vi "Receive DS Packet.vi"(0 "Recv Socket":refnum<k16>, 5 "Log User Data":bool) -> (2 "New Dashboard Data":bool, 3 "Battery":sgl, 4 "Error Strings":string, 6 "Driver Station":T1, 8 "Robot IP Address":string="10.0.0.2", 10 "Status":T3, 12 "Camera IP Address":string="10.0.0.2", 13 "Low Priority User Data":string, 14 "High Priority User Data":string, 15 "Error":T2)   [LabVIEW 2012]
uses:
  DStoPCPacketTypeDef.ctl
panel:
  out "CRC":string
  out "Team ID":u16
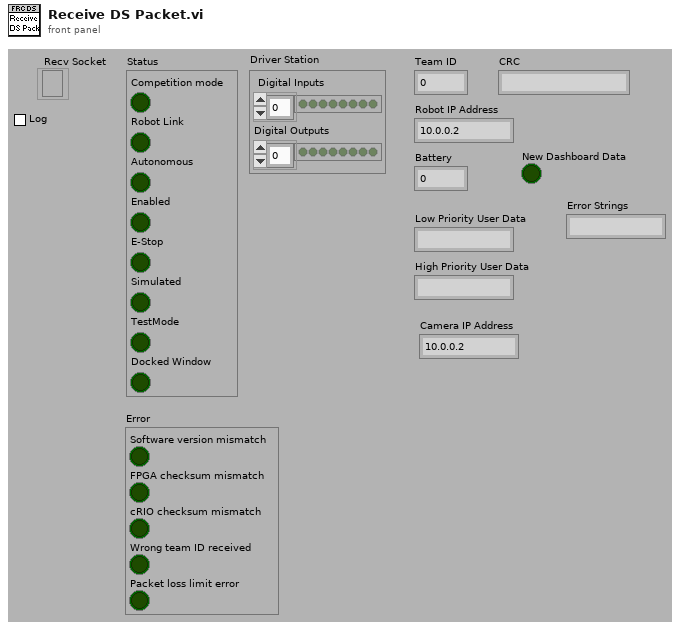
[diagram p1: front panel]
types:
  T1 = cluster{"Digital Inputs":bool[], "Digital Outputs":bool[]}
  T2 = cluster{"Software version mismatch":bool, "FPGA checksum mismatch":bool, "cRIO checksum mismatch":bool, "Wrong team ID received":bool, "Packet loss limit error":bool}
  T3 = cluster{"Competition mode":bool, "Robot Link":bool, "Autonomous":bool, "Enabled":bool, "E-Stop":bool, "Simulated":bool, "TestMode":bool, "Docked Window":bool}
  T4 = typedef "DStoPCPacketTypeDef.ctl" = cluster{"Packet Index":u16, "Digital Inputs":u8, "Digital Out":u8, "Battery":u16, "Status":u8, "Error":u8, "Team ID":u16, "VersionMonth1":u8, "VersionMonth2":u8, "VersionDay1":u8, "VersionDay2":u8, "VersionYear1":u8, "VersionYear2":u8, "Revision1":u8, "Revision2":u8, "Robot IP":u32, "UnusedBuffer 2":u8, "ExtraModeFlags":u8, "Reply Packet #":u16}
  T5 = cluster{"Boolean array":bool[], "Boolean array":bool[]}
  T6 = cluster{"Boolean array[0]":bool, "Boolean array[1]":bool, "Boolean array[2]":bool, "Boolean array[3]":bool, "Boolean array[4]":bool, "Boolean array[5]":bool, "Boolean array[6]":bool, "Boolean array[7]":bool}
  T7 = cluster{"Boolean array[0]":bool, "Boolean array[1]":bool, "Boolean array[4]":bool, "Boolean array[5]":bool, bool, bool, bool, bool}
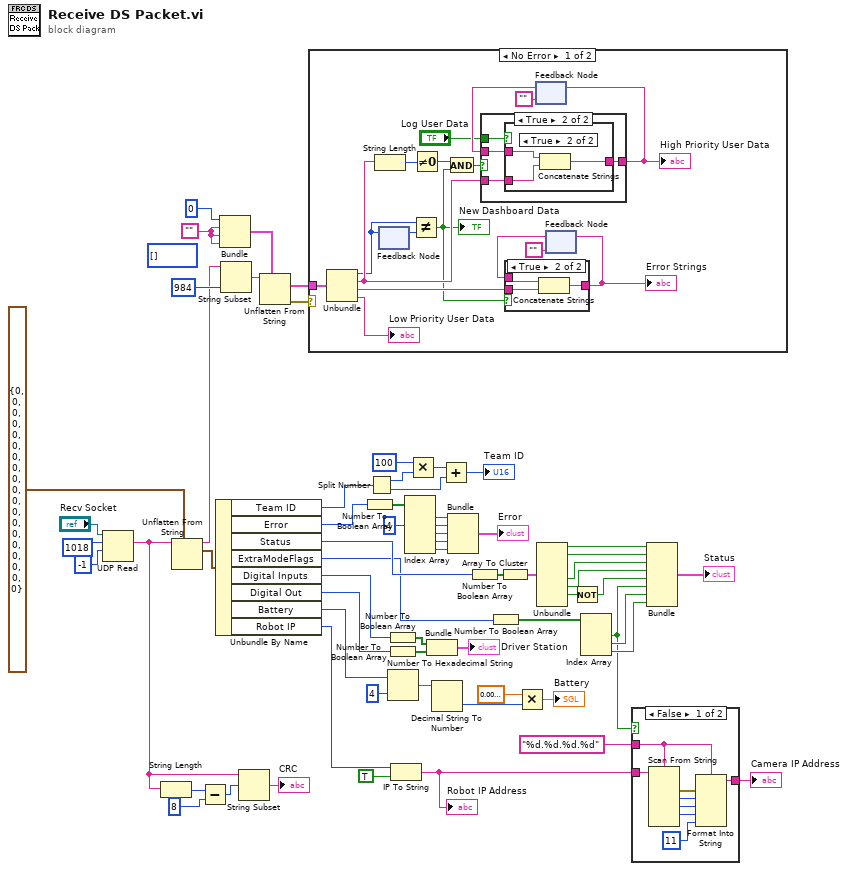
[diagram p0: block diagram]
diagram:
  (unwired) u8[] []
  w10 = ""
  n1 = UDP Read(connection ID="Recv Socket", max size (548)=1018 ("bytes to read"), timeout ms (25000)=-1) -> (data out=w30:string)  [unwired: 1 in, 4 out]
  n2 = String Length(string=w30) -> (length=w42:i32)
  n3 = Unflatten From String(type=T4 {"Packet Index"=0, "Digital Inputs"=0, "Digital Out"=0, "Battery"=0, "Status"=0, "Error"=0, "Team ID"=0, "VersionMonth1"=0, "VersionMonth2"=0, "VersionDay1"=0, "VersionDay2"=0, "VersionYear1"=0, "VersionYear2"=0, "Revision1"=0, "Revision2"=0, "Robot IP"=0, "UnusedBuffer 2"=0, "ExtraModeFlags"=0, "Reply Packet #"=0} ("Cluster"), binary string=w30) -> (rest of the binary string=w43:string, value=w64:T4)  [unwired: 1 in, 3 out]
  n4 = Subtract(x=w42, y=8) -> (x-y=w40:i32)
  n5 = Unbundle By Name(w64) -> ("Team ID"=w46:u16, "Error"=w55:u8, "Status"=w63:u8, "ExtraModeFlags"=w9:u8, "Digital Inputs"=w18:u8, "Digital Out"=w17:u8, "Battery"=w37:u16, "Robot IP"=w1:u32)
  n6 = Bundle(u8 0, w10, w10, w10) -> (w14:cluster{u8, string, string, string})  [unwired: 1 out]
  n7 = String Subset(string=w43, length (rest)=984 ("length (rest)")) -> (substring=w19:string)  [unwired: 1 out]
  n8 = String Subset(string=w30, offset (0)=w40) -> (substring=→"CRC":string)  [unwired: 1 out]
  n9 = Unflatten From String(type=w14, binary string=w19) -> (value=w12:cluster{u8, string, string, string}, error out=w11:errorcluster)  [unwired: 1 in, 3 out]
  n10 = case shown="No Error" w11 {
    tunnel: w12 -> [w78 _]
    frame No Error {
      n11 = Unbundle(w78) -> (w69:u8, w70:string, w76:string, →"Low Priority User Data":string)
      n12 = String Length(string=w70) -> (length=w71:i32)
      n13 = feedback-in #1(w69) -> ()
      n14 = feedback #1() -> (w68:u8)  [unwired: 1 out]
      n15 = Not Equal?(x=w69, y=w68) -> (x != y?=w67:bool)
      "New Dashboard Data" <- w67
      n16 = Not Equal To 0?(x=w71) -> (x != 0?=w72:bool)
      n17 = And(x=w72, y=w67) -> (x .and. y?=w73:bool)
      n18 = feedback #2("") -> (w79:string)
      n19 = case shown="True" w73 {
        tunnel: w70 -> [_ w90]
        tunnel: [w86 w89] -> w65
        tunnel: w79 -> [w86 w88]
        tunnel: "Log User Data" -> [_ w87]
        frame False {
        }
        frame True {
          n20 = case shown="True" w87 {
            tunnel: w90 -> [w91 w94]
            tunnel: [w91 w93] -> w89
            tunnel: w88 -> [_ w92]
            frame False {
            }
            frame True {
              n21 = Concatenate Strings(w92, w94) -> (w93:string)
            }
          }
        }
      }
      "High Priority User Data" <- w65
      n22 = feedback-in #2(w65) -> ()
      n23 = feedback #3("") -> (w81:string)
      n24 = case shown="True" w67 {
        tunnel: [w82 w85] -> w66
        tunnel: w81 -> [w82 w84]
        tunnel: w76 -> [_ w83]
        frame False {
        }
        frame True {
          n25 = Concatenate Strings(w84, w83) -> (w85:string)
        }
      }
      "Error Strings" <- w66
      n26 = feedback-in #3(w66) -> ()
    }
    frame Error {
    }
  }
  n27 = Number To Boolean Array(number=w55) -> (Boolean array=w26:bool[])
  n28 = Split Number(x=w46) -> (hi(x)=w52:u8, lo(x)=w49:u8)
  n29 = Number To Boolean Array(number=w18) -> (Boolean array=w15:bool[])
  n30 = Number To Boolean Array(number=w17) -> (Boolean array=w16:bool[])
  n31 = Number To Hexadecimal String(1:i16 4 ("width (-)"), 2:w37) -> (0:w36:string)
  n32 = IP To String(1:TRUE ("dot notation? (F)"), 2:w1) -> (0:w3:string)
  "Robot IP Address" <- w3
  n33 = Index Array(array=w26, index #2=4 ("index")) -> (element #1=w20:bool, element #2=w21:bool, element #3=w22:bool, element #4=w23:bool, element #5=w24:bool)  [unwired: 4 in]
  n34 = Multiply(x=u16 100, y=w52) -> (x*y=w50:u16)
  n35 = Bundle("Boolean array"=w15, "Boolean array"=w16) -> (→"Driver Station":T5)  [unwired: 1 out]
  n36 = Decimal String To Number(string=w36) -> (number=w34:i32)  [unwired: 3 out]
  n37 = Add(x=w50, y=w49) -> (x+y=→"Team ID":u16)
  n38 = Bundle(w20, w21, w22, w23, w24) -> (→"Error":cluster{bool, bool, bool, bool, bool})  [unwired: 1 out]
  n39 = Number To Boolean Array(number=w63) -> (Boolean array=w62:bool[])
  n40 = Number To Boolean Array(number=w9) -> (Boolean array=w8:bool[])
  n41 = Array To Cluster(array=w62) -> (cluster=w60:T6)
  n42 = Multiply(x=sgl 0.01, y=w34) -> (x*y=→"Battery":sgl)
  n43 = Unbundle(w60) -> ("Boolean array[0]"=w59:bool, "Boolean array[1]"=w58:bool, "Boolean array[4]"=w57:bool, "Boolean array[5]"=w56:bool, "Boolean array[6]"=w54:bool)  [unwired: 3 out]
  n44 = Not(x=w54) -> (.not. x?=w53:bool)
  n45 = Index Array(array=w8) -> (element #1=w4:bool, element #2=w7:bool, element #3=w6:bool)  [unwired: 3 in]
  n46 = case shown="False" w4 {
    tunnel: [w97 w103] -> w5
    tunnel: w3 -> [w96 w103]
    tunnel: "%d.%d.%d.%d" ("format string") -> [w95 _]
    frame False {
      n47 = Scan From String(format string=w95, input string=w96) -> (error out=w99:errorcluster, output 1=w100:i32, output 2=w101:i32, output 3=w102:i32)  [unwired: 2 in, 7 out]
      n48 = Format Into String(format string=w95, error in=w99, w100, w101, w102, 11 ("IP Suffix:")) -> (resulting string=w97:string)  [unwired: 1 in, 1 out]
    }
    frame True {
    }
  }
  "Camera IP Address" <- w5
  n49 = Bundle("Boolean array[0]"=w59, "Boolean array[1]"=w58, "Boolean array[4]"=w57, "Boolean array[5]"=w56, w53, w4, w7, w6) -> (→"Status":T7)  [unwired: 1 out]
